vi "SVPO Peak Level (1 Ch DBL WDT) with IC.vi"(6 "restart averaging? (F)":bool, 8 "initial conditions":T1={"historical max"=-inf, "historical min"=inf, "cumulative size"=0, "timestamp"=timestamp(0 s since 1904-01-01)}, 11 "scaled signal [EU]":waveform(dbl)={"t0"=timestamp(0 s since 1904-01-01), "dt"=0.0, "Y"=[]}) -> (0 "final conditions":T1, 1 "minimum level [EU]":dbl=nan, 2 "maximum level [EU]":dbl=nan, 3 "peak level [EU]":dbl=nan, 4 "duration [s]":dbl, 5 "timestamp":timestamp)   [LabVIEW 2017, in "SoundVib_VibrationLevel.lvlib"]
doc: "Uses a peak detector and computes the level of scaled time waveform signals and scaled array signals. <B>scaled signal [EU]</B> should have a zero DC component. You can attenuate the DC component with hardware AC-coupling filters and with software high-pass filters. Use this VI on embedded targets that have limited computational resources. Wire data to the scaled signal [EU] input to determine the polymorphic instance to use or manually select the instance."
uses:
  <vilib>/addons/Sound and Vibration/svt_Level/SoundVib_VibrationLevel.lvlib
  <vilib>/addons/_NISVFA/_Shared subVIs/Controls/svc_Peak Level State.ctl
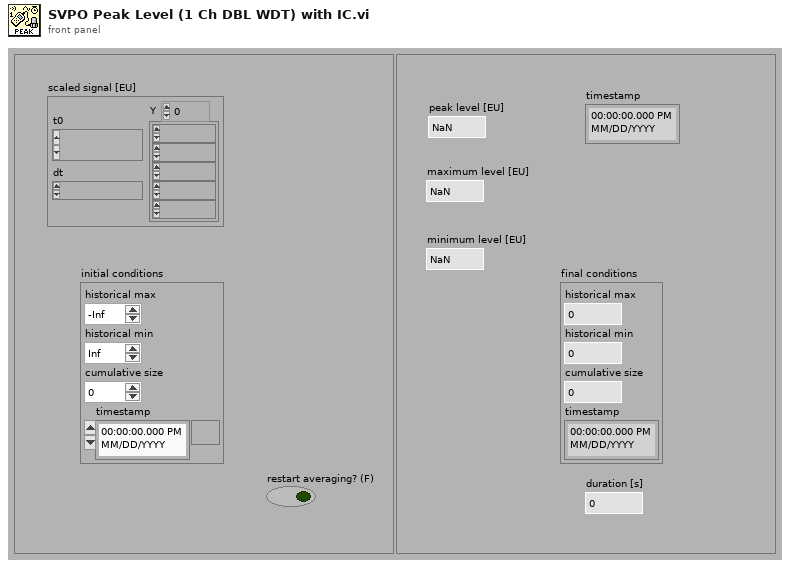
[diagram p1: front panel]
types:
  T1 = typedef "svc_Peak Level State.ctl" = cluster{"historical max":dbl, "historical min":dbl, "cumulative size":u64, "timestamp":timestamp}
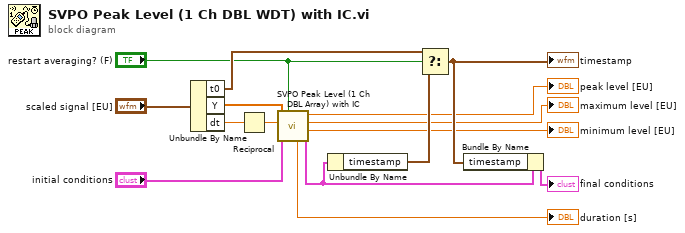
[diagram p0: block diagram]
diagram:
  n1 = Unbundle By Name("scaled signal [EU]") -> ("t0"=w14:timestamp, "Y"=w11:dbl[], "dt"=w12:dbl)
  n2 = Reciprocal(x=w12) -> (1/x=w13:dbl)
  n3 = call <vilib>:"SVPO Peak Level (1 Ch DBL Array) with IC.vi"("restart averaging? (F)"="restart averaging? (F)", "initial conditions"="initial conditions", "sampling rate [Hz]"=w13, "scaled signal [EU]"=w11) -> ("final conditions"=w1:T1, "minimum level [EU]"=→"minimum level [EU]":dbl, "maximum level [EU]"=→"maximum level [EU]":dbl, "peak level [EU]"=→"peak level [EU]":dbl, "duration [s]"=→"duration [s]":dbl)  [unwired: 3 in]
  n4 = Unbundle By Name(w1) -> ("timestamp"=w9:timestamp)
  n5 = Select(t=w14, s="restart averaging? (F)", f=w9) -> (s? t:f=w8:timestamp)
  "timestamp" <- w8
  n6 = Bundle By Name(cluster=w1, "timestamp"=w8) -> (→"final conditions":T1)
